vi "Parse for stabilization power.vi"(8 "error in (no error)":errorcluster, 10 "data":waveform(dbl)[](array[waveform])) -> (0 "error out":errorcluster, 2 "Power Values":T1, 3 "active power [W]":dbl)   [LabVIEW 2013]
uses:
  Controls/Power Values.ctl
  <vilib>/addons/Electrical Power/Basic/Measurement/subVIs/basic_Power Value.ctl
  <vilib>/addons/Electrical Power/Basic/Measurement/Power (N Channels).vi
  <vilib>/addons/Electrical Power/Basic/NI_EP_Basic.lvlib
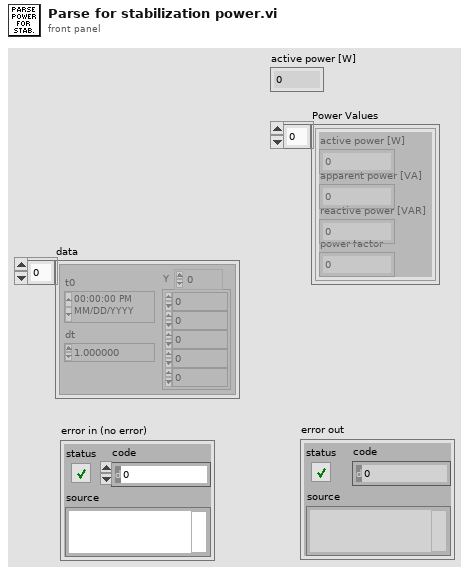
[diagram p1: front panel]
types:
  T1 = typedef "Power Values.ctl" = T2[]
  T2 = typedef "NI_EP_Basic.lvlib/basic_Power Value.ctl" = cluster{"active power [W]":dbl, "apparent power [VA]":dbl, "reactive power [VAR]":dbl, "power factor":dbl}
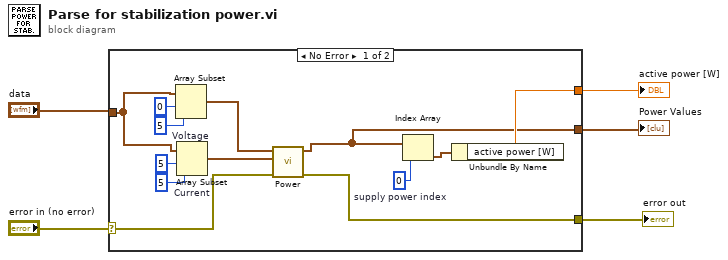
[diagram p0: block diagram]
diagram:
  n1 = case shown="No Error" "error in (no error)" {
    selector: "error in (no error)" -> [w9 w19]
    tunnel: [w18 _] -> w1
    tunnel: "data" -> [w17 _]
    tunnel: [w6 _] -> w4
    tunnel: [w8 w19] -> w2
    frame No Error {
      w16 = 0  # supply power index
      n2 = Array Subset "Voltage"(array=w17, index=0, length=5) -> (w14:waveform(dbl)[])
      n3 = Array Subset "Current"(array=w17, index=5, length=5) -> (w15:waveform(dbl)[])
      n4 = call-poly <vilib>:"Power.vi"("error in (no error)"=w9, "current waveforms"=w15, "voltage waveforms"=w14) -> ("error out"=w8:errorcluster, "power values"=w6:T2[])  [unwired: 7 in]
      n5 = Index Array(array=w6, index=w16) -> (element=w7:T2)
      n6 = Unbundle By Name(w7) -> ("active power [W]"=w18:dbl)
    }
    frame Error {
    }
  }
  "active power [W]" <- w1
  "Power Values" <- w4
  "error out" <- w2
